vi "gu_codepoint_array_to_string.vi"(8 "error in":errorcluster, 11 "Codepoint Array":i32[](array[numeric]) format="%04x") -> (0 "error out":errorcluster, 3 "Encoded String":T1)   [LabVIEW 2020, in "G-Unicode.lvlib"]
uses:
  G-Unicode.lvlib
  Types/Encoded UTF-8 String.ctl
  Memory/Copy String.vi/4d47babd-4a2d-4eb7-b91b-7e707d692665.vi
  gu_free.vi
  <vilib>/Utility/error.llb/Error Cluster From Error Code.vi
  lib/g_unicode_32.dll
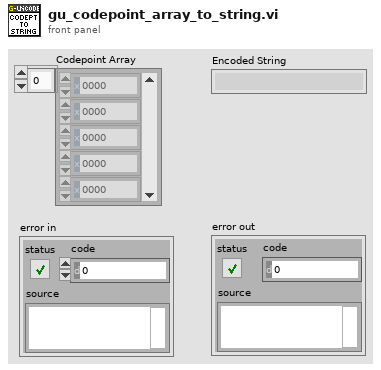
[diagram p1: front panel]
types:
  T1 = typedef "G-Unicode.lvlib/Encoded UTF-8 String.ctl" = string
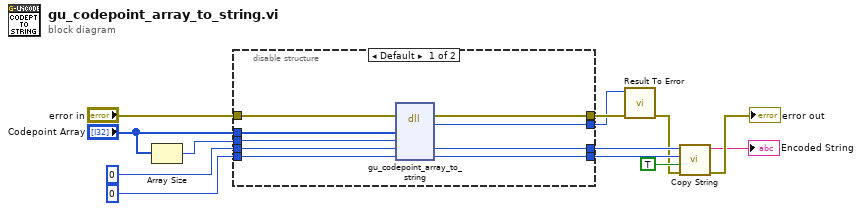
[diagram p0: block diagram]
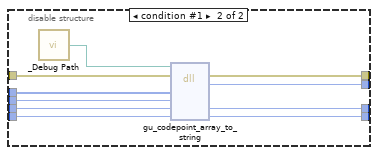
[diagram p2: hidden frame]
diagram:
  n1 = Array Size(array="Codepoint Array") -> (size(s)=w2:i32)
  n2 = disable-structure shown="Default" {
    disable-tunnel: "Codepoint Array" -> [w15 w25]
    disable-tunnel: "error in" -> [w22 w32]
    disable-tunnel: [w21 w31] -> w12
    disable-tunnel: [w20 w30] -> w10
    disable-tunnel: [w19 w29] -> w9
    disable-tunnel: [w18 w28] -> w11
    disable-tunnel: i64 0 ("codepoint_array") -> [w17 w27]
    disable-tunnel: i64 0 ("codepoint_array_size") -> [w16 w26]
    disable-tunnel: w2 -> [w14 w24]
    frame condition #0 (active) {
      n3 = dll-call lib="C:/github/dataflowg/g-unicode/src/LabVIEW/G-Unicode/lib/g_unicode_*.*" fn="gu_codepoint_array_to_string"(error in=w22, "codepoint_array"=w15, "codepoint_array_size"=w14, "str_pointer"=w17, "str_size"=w16) -> (error out=w21:errorcluster, "result"=w18:i32, "str_pointer"=w20:i64, "str_size"=w19:i32)  [unwired: 4 in, 1 out]
    }
    frame condition #1 {
      n4 = call "_Debug Path.vi"() -> ("Debug Path"=w23:path)
      n5 = dll-call lib="?" fn="gu_codepoint_array_to_string"(path in=w23, error in=w32, "codepoint_array"=w25, "codepoint_array_size"=w24, "str_pointer"=w27, "str_size"=w26) -> (error out=w31:errorcluster, "result"=w28:i32, "str_pointer"=w30:i64, "str_size"=w29:i32)  [unwired: 3 in, 1 out]
    }
  }
  n6 = call "Result To Error.vi"("error in (no error)"=w12, "Result Code"=w11) -> ("error out"=w7:errorcluster)  [unwired: 9 in]
  n7 = call "Copy String.vi"("error in"=w7, "free (F)"=TRUE, "size"=w9, "pointer"=w10) -> ("error out"=→"error out":errorcluster, "string"=→"Encoded String":string)  [unwired: 6 in]
